vi "Main.vi"(0 "A":dbl, 5 "B":dbl, 7 "Stop":bool, 11 "Error in":errorcluster, 13 "Operation":T1) -> (4 "C":dbl, 15 "Error out":errorcluster)   [LabVIEW 2020, in "Simple calculator.lvlib"]
doc: "This Vi is used to implement overriding in oops in labview"
uses:
  Simple calculator.lvlib
  Typedefs/Math Operations.ctl
  Math Operations/Math Operations.lvclass
  Math Operations/Add/Add.lvclass
  C:/Users/khishore.kumar/Khishore/labview_tips_2024/src/Assignment 24/Math Operations/Math Operations.lvclass
  Math Operations/Subtract/Subtract.lvclass
  Math Operations/Multiply/Multiply.lvclass
  Math Operations/Divide/Divide.lvclass
panel:
  # "MATH OPERATIONS"
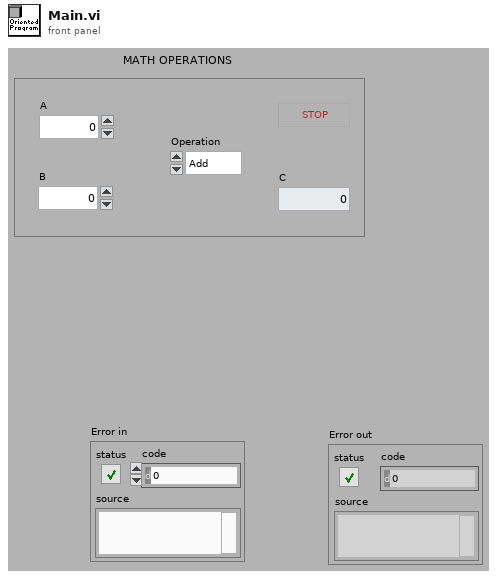
[diagram p1: front panel]
types:
  T1 = typedef "Simple calculator.lvlib/Math Operations.ctl" = enum16{"Add", "Subtract", "Multiply", "Divide"}
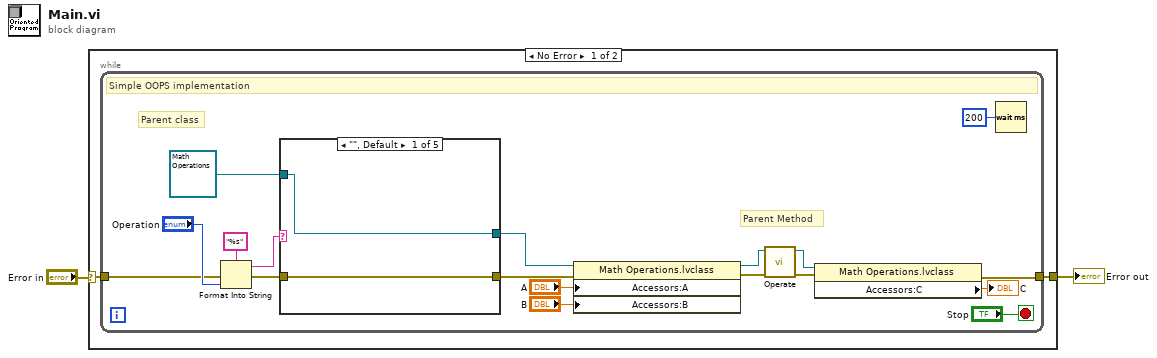
[diagram p0: block diagram]
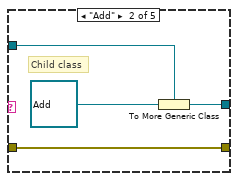
[diagram p2: hidden frame]
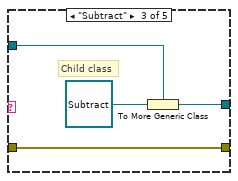
[diagram p3: hidden frame]
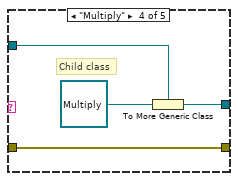
[diagram p4: hidden frame]
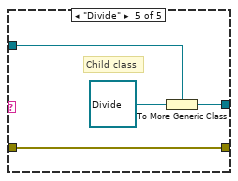
[diagram p5: hidden frame]
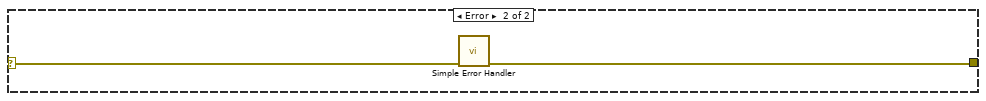
[diagram p6: hidden frame]
diagram:
  n1 = case shown="No Error" "Error in" {
    selector: "Error in" -> [w3 w42]
    tunnel: [w4 w41] -> w2
    frame No Error {
      n2 = while {
        tunnel: w3 -> [w6]
        tunnel: [w18] -> w4
        stop <- "Stop" stop-if-true
        # "Parent Method"
        # "Parent class"
        # "Simple OOPS implementation"
        n3 = Format Into String(format string="%s", error in=w6, "Operation") -> (resulting string=w7:string, error out=w5:errorcluster)  [unwired: 1 in]
        n4 = case shown="\"\", Default" w7 {
          tunnel: w5 -> [w24 w26 w32 w36 w40]
          tunnel: [w24 w26 w32 w36 w40] -> w15
          tunnel: refnum<class "Math Operations.lvclass"> refnum ("Math Operations.lvclass") -> [w23 w28 w29 w33 w37]
          tunnel: [w23 w27 w30 w34 w38] -> w16
          frame "", Default {
          }
          frame "Add" {
            # "Child class"
            n5 = To More Generic Class(target class=w28, reference=refnum<class "Add.lvclass"> refnum ("Add.lvclass")) -> (generic class reference=w27:refnum<class "Math Operations.lvclass">)
          }
          frame "Subtract" {
            # "Child class"
            n6 = To More Generic Class(target class=w29, reference=refnum<class "Subtract.lvclass"> refnum ("Subtract.lvclass")) -> (generic class reference=w30:refnum<class "Math Operations.lvclass">)
          }
          frame "Multiply" {
            # "Child class"
            n7 = To More Generic Class(target class=w33, reference=refnum<class "Multiply.lvclass"> refnum ("Multiply.lvclass")) -> (generic class reference=w34:refnum<class "Math Operations.lvclass">)
          }
          frame "Divide" {
            # "Child class"
            n8 = To More Generic Class(target class=w37, reference=refnum<class "Divide.lvclass"> refnum ("Divide.lvclass")) -> (generic class reference=w38:refnum<class "Math Operations.lvclass">)
          }
        }
        n9 = property class="Math Operations.lvclass"(reference=w16, error in=w15, "Accessors:A"="A", "Accessors:B"="B") -> (reference out=w13:refnum<class "Math Operations.lvclass">, error out=w14:errorcluster)
        n10 = call-dynamic "Operate.vi"("error in (no error)"=w14, "Math Operations in"=w13) -> ("error out"=w12:errorcluster, "Math Operations out"=w11:refnum<class "Math Operations.lvclass">)  [unwired: 8 in]
        n11 = property class="Math Operations.lvclass"(reference=w11, error in=w12) -> (error out=w18:errorcluster, "Accessors:C"=→"C":dbl)  [unwired: 1 out]
        n12 = Wait (ms)(milliseconds to wait=u32 200) -> ()  [unwired: 1 out]
      }
    }
    frame Error {
      n13 = call <vilib>:"Simple Error Handler.vi"("error in (no error)"=w42) -> ("error out"=w41:errorcluster)  [unwired: 4 in, 4 out]
    }
  }
  "Error out" <- w2
